vi "Read Discret Registers.vi"(0 "Refnum in":refnum<visa-resource-name>, 1 "startReg":u16, 2 "Quantity":u16=1, 5 "Mode":T1, 11 "error in (no error)":errorcluster, 12 "Enable":bool) -> (4 "Refnum Out":refnum<visa-resource-name>, 6 "ModeOut":T1, 8 "Discret Registers":bool[](array[boolean]), 15 "error out":errorcluster)   [LabVIEW 2020]
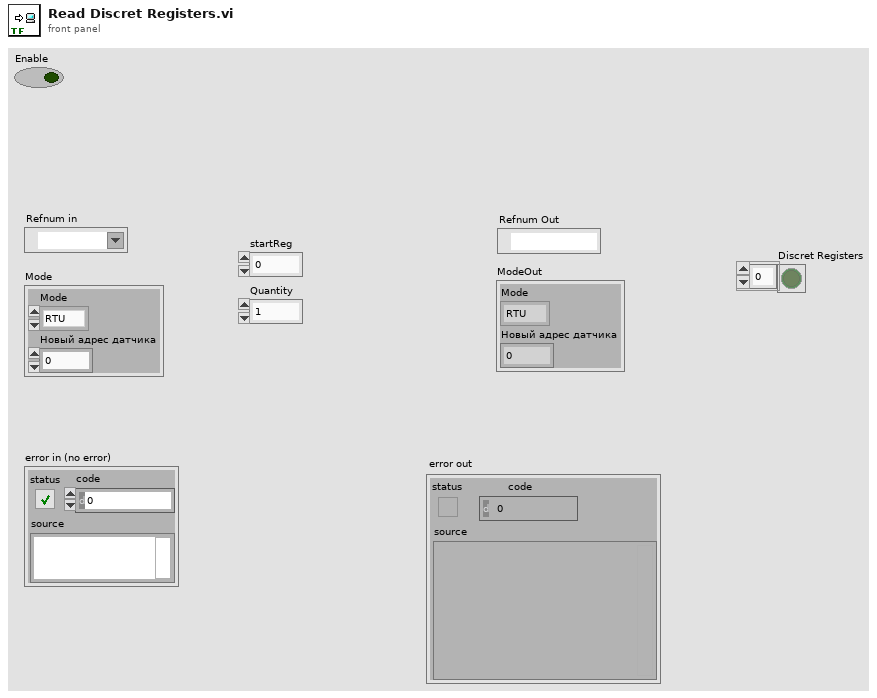
[diagram p1: front panel]
types:
  T1 = cluster{"Mode":enum16{"RTU", "ASCII"}, "Новый адрес датчика":u16}
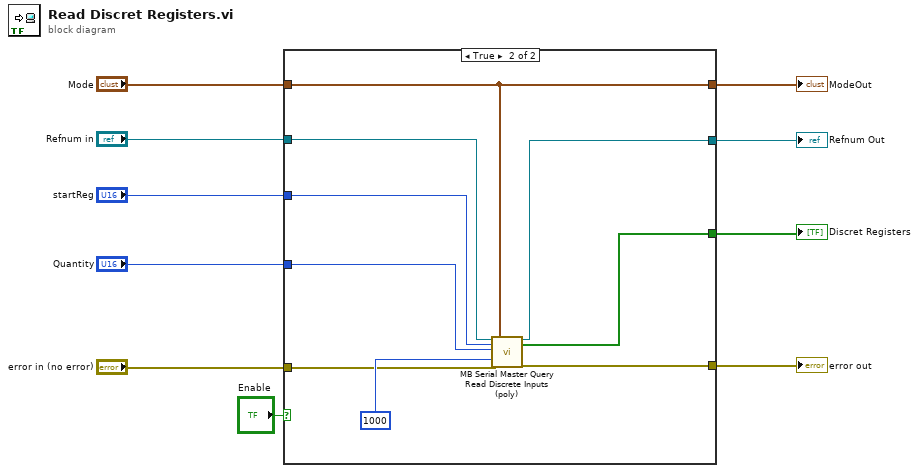
[diagram p0: block diagram]
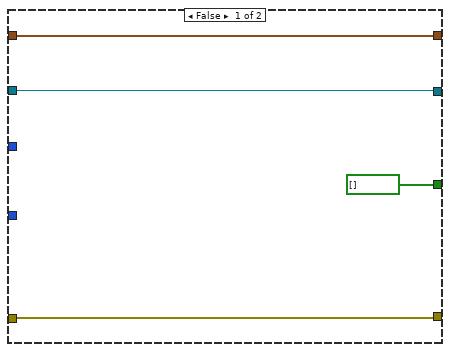
[diagram p2: hidden frame]
diagram:
  n1 = case shown="True" "Enable" {
    tunnel: "Mode" -> [w13 w18]
    tunnel: "error in (no error)" -> [w14 w22]
    tunnel: "Refnum in" -> [w12 w17]
    tunnel: "startReg" -> [_ w21]
    tunnel: "Quantity" -> [_ w20]
    tunnel: [w14 w19] -> w6
    tunnel: [w13 w18] -> w4
    tunnel: [w12 w16] -> w3
    tunnel: [bool[] [] ("Holding Registers") w15] -> w1
    frame False {
    }
    frame True {
      n2 = call <vilib>:"MB Serial Master Query Read Discrete Inputs (poly).vi"("VISA resource name"=w17, "Starting Address"=w21, "Quantity"=w20, "Timeout"=u32 1000, "error in"=w22, "Serial Parameters"=w18) -> ("VISA resource name out"=w16:refnum<visa-resource-name>, "Discrete Inputs"=w15:bool[], "error out"=w19:errorcluster)  [unwired: 10 in, 1 out]
    }
  }
  "error out" <- w6
  "ModeOut" <- w4
  "Refnum Out" <- w3
  "Discret Registers" <- w1
